vi "Read Name core.vi"(11 "Build Item in":refnum<class "Apply VIPC Step.lvclass">) -> (2 "Name":string)   [LabVIEW 2019, in "VIPM.lvlib" / "Apply VIPC Step.lvclass"]
doc: "Gets the name for the build step\n\nCopyright: MGI 2016\nAuthor: Derek Trepanier"
uses:
  Apply VIPC Step.lvclass
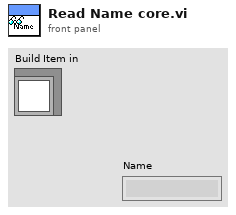
[diagram p1: front panel]
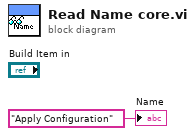
[diagram p0: block diagram]
diagram:
  "Name" <- "Apply Configuration" ("Name")
